vi "Update DatabaseO.vi"(2 "DC_SN":string, 4 "OscData":string, 8 "TimeStart":string, 9 "connection information":path) -> ()   [LabVIEW 2024]
uses:
  <vilib>/addons/database/NI_Database_API.lvlib
  <vilib>/addons/database/_DB Variant To Data/Database Variant To Data.xnode
  <vilib>/addons/database/Connection.llb/DB Tools Open Connec (Path).vi
  <vilib>/addons/database/Connection.llb/Conn Execute.vi
  <vilib>/addons/database/Recordset.llb/Rec Destroy - Connection.vi
panel:
  out "Time Measured":string
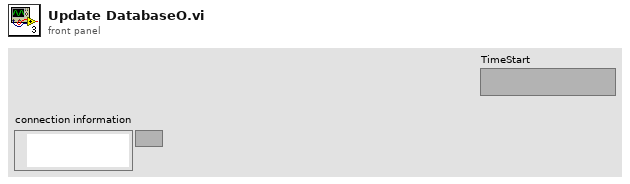
[diagram p1: front panel]
types:
  T1 = typedef "NI_Database_API.lvlib/Conn ObjectReference.ctl" = refnum<k1>
  T2 = typedef "NI_Database_API.lvlib/Rec ObjectReference.ctl" = refnum<k1>
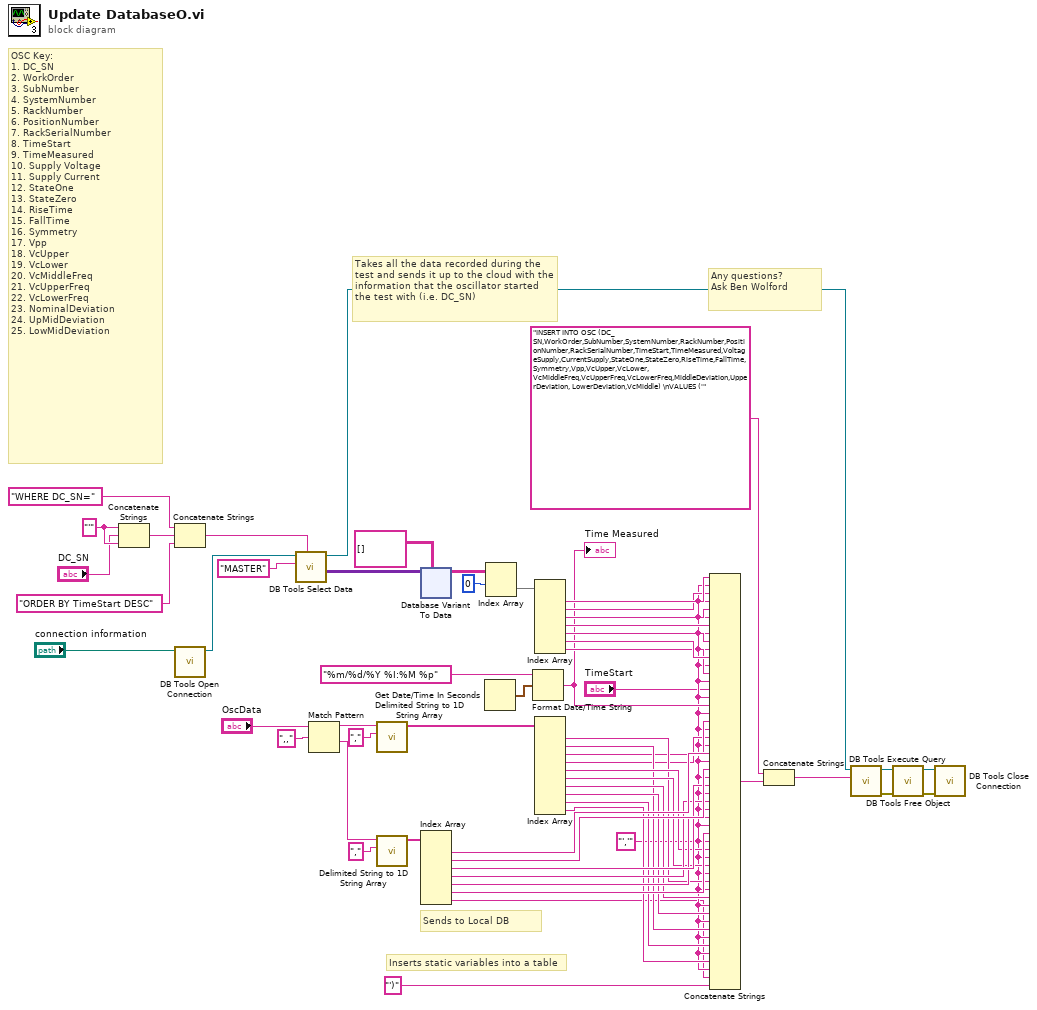
[diagram p0: block diagram]
diagram:
  w17 = "'" ("string")
  w23 = "','"
  # "Takes all the data recorded during the test and sends it up to the cloud with the information that the oscillator started the test with (i.e. DC_SN)"
  # "Sends to Local DB"
  # "Inserts static variables into a table"
  # "OSC Key:\n1. DC_SN\n2. WorkOrder\n3. SubNumber\n4. SystemNumber\n5. RackNumber\n6. PositionNumber\n7. RackSerialNumber\n8. TimeStart\n9. TimeMeasured\n10. Supply Voltage\n11. Supply Current\n12. StateOne\n13. StateZero\n14. RiseTime\n15. FallTime\n16. Symmetry\n17. Vpp\n18. VcUpper\n19. VcLower\n20. VcMiddleFreq\n21. VcUpperFreq\n22. VcLowerFreq\n23. NominalDeviation\n24. UpMidDeviation\n25. LowMidDeviation"
  # "Any questions? \nAsk Ben Wolford"
  n1 = Concatenate Strings(w17, "DC_SN", w17) -> (w16:string)
  n2 = Concatenate Strings("WHERE DC_SN=" ("SQL Query"), w16, "ORDER BY TimeStart DESC" ("string")) -> (w10:string)
  n3 = call-poly <vilib>:"DB Tools Open Connection.vi"("connection information"="connection information") -> ("connection reference"=w13:T1)  [unwired: 7 in, 1 out]
  n4 = call <vilib>:"DB Tools Select Data.vi"("condition"=w10, "table"="MASTER", "connection reference"=w13) -> ("data"=w14:variant[][], "connection reference out"=w2:T1)  [unwired: 3 in, 1 out]
  n5 = Match Pattern(string="OscData", regular expression=",,") -> (before substring=w46:string, after substring=w44:string)  [unwired: 1 in, 2 out]
  n6 = call <vilib>:"Delimited String to 1D String Array.vi"("delimiter"=",", "delimited string"=w46) -> ("string array"=w36:string[])  [unwired: 9 in]
  n7 = call <vilib>:"Delimited String to 1D String Array.vi"("delimiter"=",", "delimited string"=w44) -> ("string array"=w43:string[])  [unwired: 9 in]
  n8 = xnode "Database Variant To Data"("database variant"=w14, "type"=string[][] []) -> ("data"=w9:string[][])  [unwired: 1 in, 1 out]
  n9 = Index Array(array=w43) -> (element #1=w42:string, element #2=w41:string, element #3=w40:string, element #4=w39:string, element #5=w38:string, element #6=w37:string, element #7=w22:string)  [unwired: 7 in]
  n10 = Get Date/Time In Seconds() -> (seconds since 1Jan1904=w58:timestamp)
  n11 = Index Array(array=w9, index (row)=0 ("disabled index (row)")) -> (element=w8:string[])  [unwired: 1 in]
  n12 = Format Date/Time String(time format string (%c)="%m/%d/%Y %I:%M %p", seconds (now)=w58) -> (date/time string=w25:string)  [unwired: 1 in]
  "Time Measured" <- w25
  n13 = Index Array(array=w8) -> (element #1=w56:string, element #2=w55:string, element #3=w54:string, element #4=w53:string, element #5=w52:string, element #6=w51:string, element #7=w50:string)  [unwired: 7 in]
  n14 = Index Array(array=w36) -> (element #1=w33:string, element #2=w30:string, element #3=w27:string, element #4=w26:string, element #5=w35:string, element #6=w34:string, element #7=w32:string, element #8=w31:string, element #9=w29:string, element #10=w28:string)  [unwired: 10 in]
  n15 = Concatenate Strings(w56, w23, w55, w23, w54, w23, w53, w23, w52, w23, w51, w23, w50, w23, "TimeStart", w23, w25, w23, w27, w23, w26, w23, w42, w23, w41, w23, w40, w23, w39, w23, w38, w23, w37, w23, w35, w23, w34, w23, w33, w23, w32, w23, w31, w23, w30, w23, w29, w23, w28, w23, w22, "')" ("string")) -> (w59:string)
  n16 = Concatenate Strings("INSERT INTO OSC (DC_SN,WorkOrder,SubNumber,SystemNumber,RackNumber,PositionNumber,RackSerialNumber,TimeStart,TimeMeasured,VoltageSupply,CurrentSupply,StateOne,StateZero,RiseTime,FallTime,Symmetry,Vpp,VcUpper,VcLower, VcMiddleFreq,VcUpperFreq,VcLowerFreq,MiddleDeviation,UpperDeviation, LowerDeviation,VcMiddle) \nVALUES ('" ("string"), w59) -> (w1:string)
  n17 = call-poly <vilib>:"DB Tools Execute Query.vi"("SQL query"=w1, "connection reference"=w2) -> ("error out"=w4:errorcluster, "recordset reference"=w3:T2)  [unwired: 6 in]
  n18 = call-poly <vilib>:"DB Tools Free Object.vi"("error in (no error)"=w4, "recordset reference"=w3) -> ("error out"=w6:errorcluster, "connection reference"=w5:T1)  [unwired: 8 in]
  n19 = call <vilib>:"DB Tools Close Connection.vi"("error in (no error)"=w6, "connection reference"=w5) -> ()  [unwired: 5 in, 1 out]
